vi "Calculate Control Position.vi"(8 "error in (no error)":errorcluster, 9 "Panel Position":T2, 10 "Panel Bound":T1, 11 "Control Bound":T1) -> (0 "error out":errorcluster, 3 "Control Position Out":T2)   [LabVIEW 2015, in "ScriptDialog.lvclass"]
uses:
  ScriptDialog.lvclass
  <vilib>/Utility/miscctls.llb/LVPositionTypeDef.ctl
  <vilib>/Utility/miscctls.llb/LVBoundsTypeDef.ctl
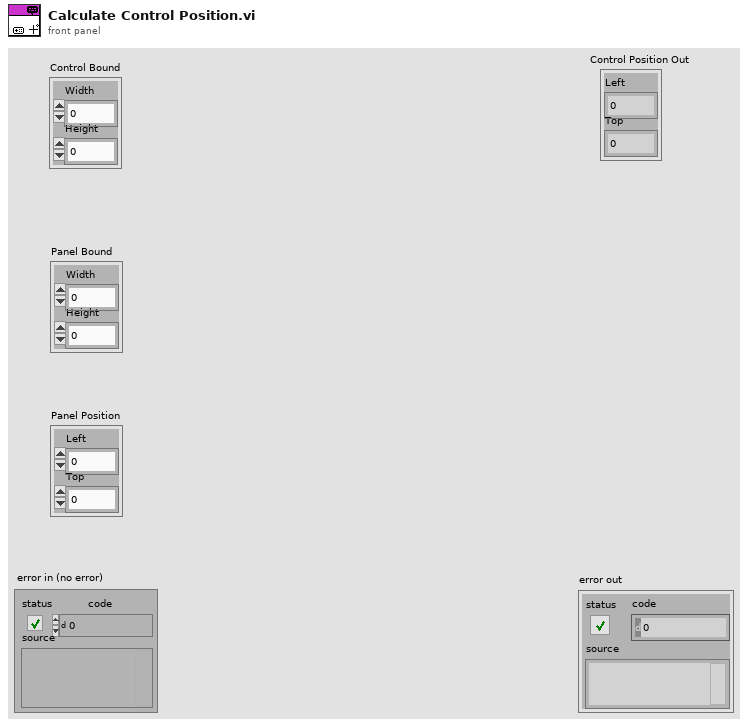
[diagram p1: front panel]
types:
  T1 = typedef "LVBoundsTypeDef.ctl" = cluster{"Width":u32, "Height":u32}
  T2 = typedef "LVPositionTypeDef.ctl" = cluster{"Left":i32, "Top":i32}
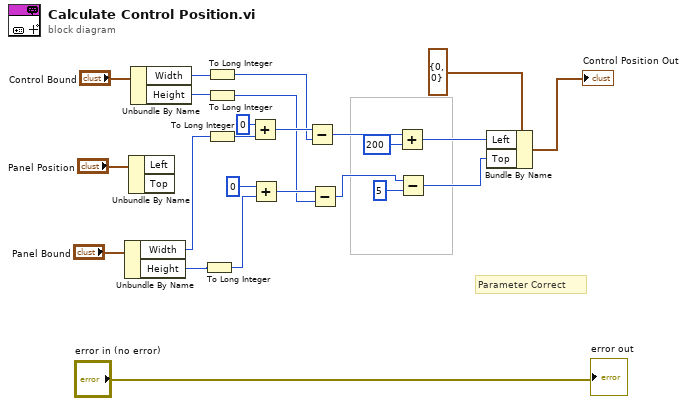
[diagram p0: block diagram]
diagram:
  # "Parameter Correct"
  n1 = Unbundle By Name("Panel Bound") -> ("Width"=w22:u32, "Height"=w20:u32)
  n2 = Unbundle By Name("Panel Position") -> ()  [unwired: 2 out]
  n3 = Unbundle By Name("Control Bound") -> ("Width"=w16:u32, "Height"=w15:u32)
  n4 = To Long Integer(number=w20) -> (32bit integer=w19:i32)
  n5 = To Long Integer(number=w16) -> (32bit integer=w14:i32)
  n6 = To Long Integer(number=w15) -> (32bit integer=w12:i32)
  n7 = To Long Integer(number=w22) -> (32bit integer=w21:i32)
  n8 = Add(x=0, y=w21) -> (x+y=w18:i32)
  n9 = Add(x=0, y=w19) -> (x+y=w13:i32)
  n10 = Subtract(x=w18, y=w14) -> (x-y=w8:i32)
  n11 = Subtract(x=w13, y=w12) -> (x-y=w5:i32)
  n12 = Add(x=w8, y=200) -> (x+y=w6:i32)
  n13 = Subtract(x=w5, y=5) -> (x-y=w3:i32)
  n14 = Bundle By Name(cluster=T2 {"Left"=0, "Top"=0} ("Control Position Out"), "Left"=w6, "Top"=w3) -> (→"Control Position Out":T2)
  "error out" <- "error in (no error)"
